vi "Init.vi"(8 "error in (no error)":errorcluster caption="entrée d'erreur (pas d'erreur)") -> (0 "error out":errorcluster caption="sortie d'erreur", 3 "L298N en sortie":refnum<class "L298N.lvclass">)   [LabVIEW 2019, in "L298N.lvclass"]
uses:
  L298N.lvclass
  L298N.lvclass/L298N.ctl
panel:
  out "élément":tag
  in  "Channel Names":tag[](array[tag])
  in  "IN4":string
  in  "IN3":string
  in  "IN2":string
  in  "IN1":string
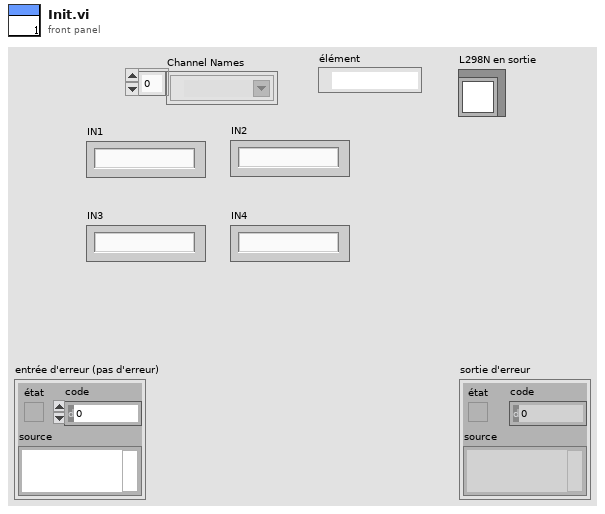
[diagram p1: front panel]
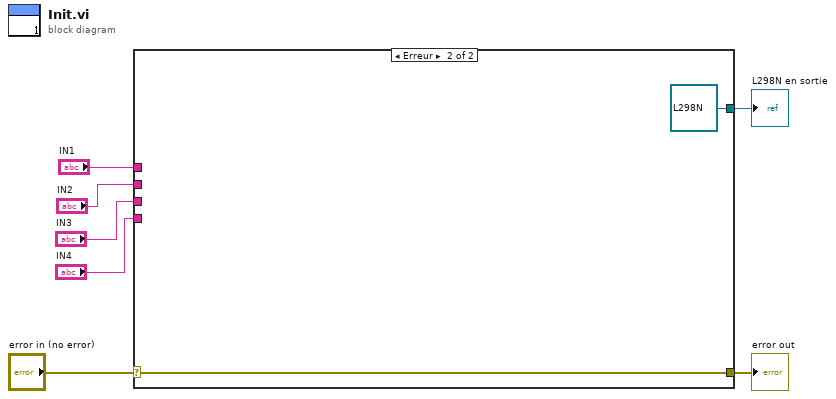
[diagram p0: block diagram]
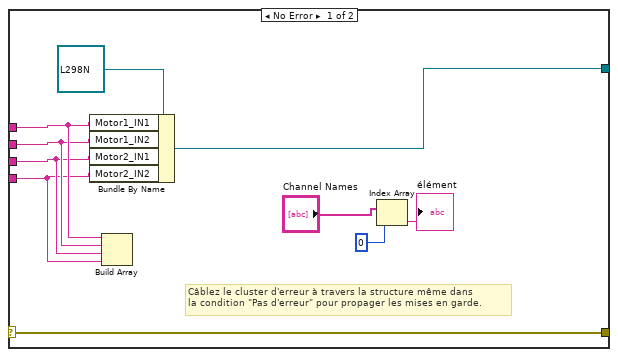
[diagram p2: hidden frame]
diagram:
  n1 = case shown="Erreur" "error in (no error)" {
    selector: "error in (no error)" -> [w17 w19]
    tunnel: [w17 w19] -> w6
    tunnel: [w16 refnum<class "L298N.lvclass"> refnum ("L298N en entrée")] -> w5
    tunnel: "IN1" -> [w15 _]
    tunnel: "IN2" -> [w14 _]
    tunnel: "IN3" -> [w13 _]
    tunnel: "IN4" -> [w12 _]
    frame No Error {
      # "Câblez le cluster d'erreur à travers la structure même dans\nla condition \"Pas d'erreur\" pour propager les mises en garde."
      n2 = Bundle By Name(cluster=refnum<class "L298N.lvclass"> refnum ("L298N en entrée"), "Motor1_IN1"=w15, "Motor1_IN2"=w14, "Motor2_IN1"=w13, "Motor2_IN2"=w12) -> (w16:refnum<class "L298N.lvclass">)
      n3 = Build Array(w15, w14, w13, w12) -> ()  [unwired: 1 out]
      n4 = Index Array(array="Channel Names", index=0 ("indice")) -> (element=→"élément":tag)
    }
    frame Error {
    }
  }
  "error out" <- w6
  "L298N en sortie" <- w5
